vi "MU Acquire MtSync Data.vi"(6 "AnyThread? (F)":bool, 8 "error in (no error)":errorcluster, 10 "numberOfSamples":u64, 11 "MUhandle":u64) -> (0 "error out (no error)":errorcluster, 2 "data":T1(array[cluster]), 3 "function return":u32)   [LabVIEW 2017, in "MU_3SL_interface.lvlib"]
uses:
  MU_3SL_interface.lvlib
  lib/MU_3SL_interface.dll
panel:
  in  "data":T2
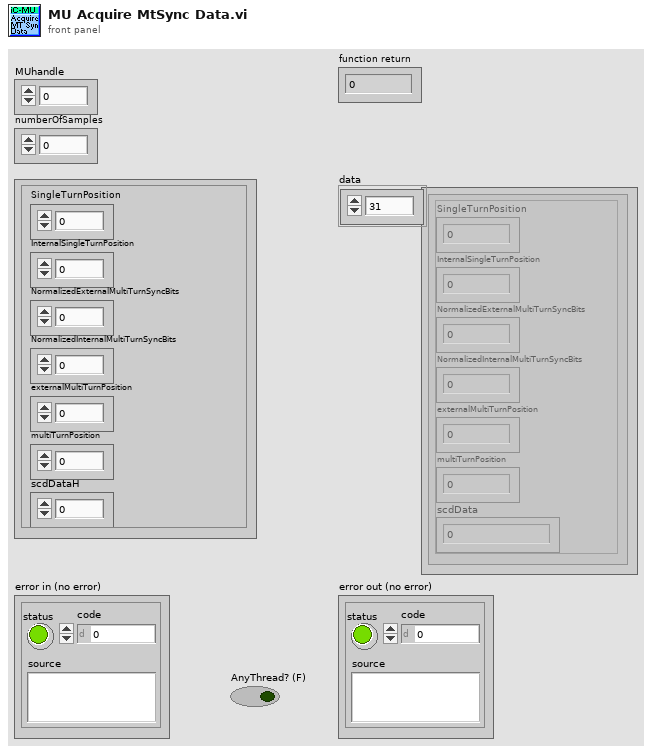
[diagram p1: front panel]
types:
  T1 = cluster{"SingleTurnPosition":u32, "InternalSingleTurnPosition":u32, "NormalizedExternalMultiTurnSyncBits":u32, "NormalizedInternalMultiTurnSyncBits":u32, "externalMultiTurnPosition":u32, "multiTurnPosition":u32, "scdData":u64}[]
  T2 = cluster{"SingleTurnPosition":u32, "InternalSingleTurnPosition":u32, "NormalizedExternalMultiTurnSyncBits":u32, "NormalizedInternalMultiTurnSyncBits":u32, "externalMultiTurnPosition":u32, "multiTurnPosition":u32, "scdDataH":u64}
  T3 = cluster{"SingleTurnPosition":u32, "InternalSingleTurnPosition":u32, "NormalizedExternalMultiTurnSyncBits":u32, "NormalizedInternalMultiTurnSyncBits":u32, "externalMultiTurnPosition":u32, "multiTurnPosition":u32, "scdDataH":u64}[]
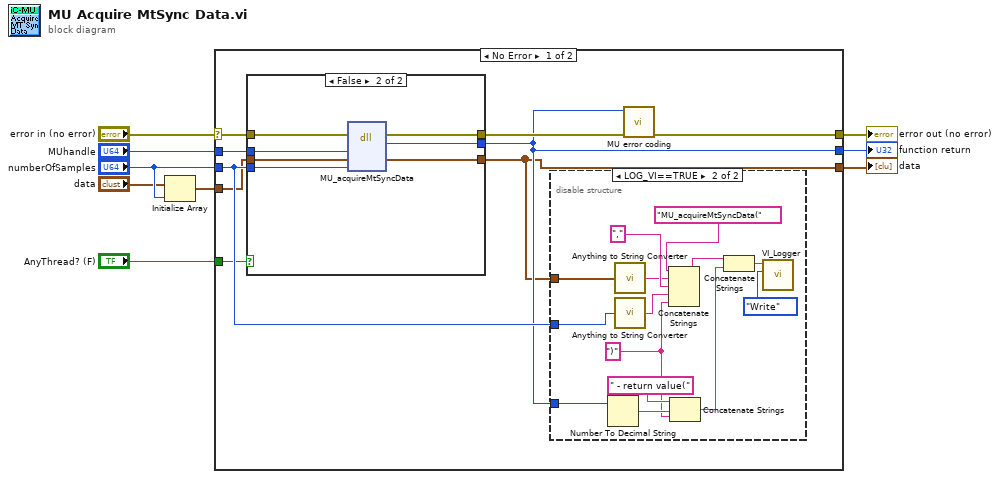
[diagram p0: block diagram]
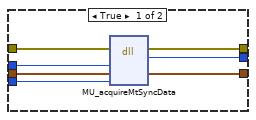
[diagram p2: hidden frame]
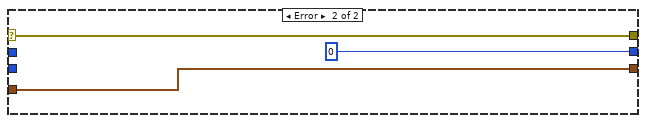
[diagram p4: hidden frame]
diagram:
  n1 = Initialize Array("data", "numberOfSamples") -> (w3:T3)
  n2 = case shown="No Error" "error in (no error)" {
    selector: "error in (no error)" -> [w15 w49]
    tunnel: [w13 u32 0] -> w9
    tunnel: "MUhandle" -> [w18 _]
    tunnel: [w16 w49] -> w7
    tunnel: "numberOfSamples" -> [w14 _]
    tunnel: w3 -> [w11 w47]
    tunnel: [w10 w47] -> w2
    tunnel: "AnyThread? (F)" -> [w12 _]
    frame No Error {
      n3 = case shown="False" w12 {
        tunnel: w18 -> [w25 w32]
        tunnel: [w24 w31] -> w17
        tunnel: w15 -> [w23 w30]
        tunnel: w11 -> [w22 w29]
        tunnel: w14 -> [w21 w28]
        tunnel: [w20 w27] -> w13
        tunnel: [w19 w26] -> w10
        frame True {
          n4 = dll-call lib="C:/Users/bes/AppData/Roaming/work/mu_9so/icsubmodules/soft_mu_3sl_master/lv_interface/lib/MU_3SL_interface**.*" fn="MU_acquireMtSyncData"(error in=w23, "MUhandle"=w25, "data"=w22, "numberOfSamples"=w21) -> (error out=w24:errorcluster, "return type"=w20:u32, "data"=w19:T3)  [unwired: 4 in, 1 out]
        }
        frame False {
          n5 = dll-call lib="C:/Users/bes/AppData/Roaming/work/mu_9so/icsubmodules/soft_mu_3sl_master/lv_interface/lib/MU_3SL_interface**.*" fn="MU_acquireMtSyncData"(error in=w30, "MUhandle"=w32, "data"=w29, "numberOfSamples"=w28) -> (error out=w31:errorcluster, "return type"=w27:u32, "data"=w26:T3)  [unwired: 4 in, 1 out]
        }
      }
      n6 = disable-structure shown="LOG_VI==TRUE" {
        disable-tunnel: w13 -> [_ w44]
        disable-tunnel: w14 -> [_ w36]
        disable-tunnel: w10 -> [_ w34]
        frame condition #0 {
        }
        frame condition #1 (active) {
          w37 = ")" ("string")
          n7 = Number To Decimal String(number=w44) -> (decimal integer string=w43:string)  [unwired: 1 in]
          n8 = call "Anything to String Converter.vi"("anything"=w34) -> ("String"=w33:string)
          n9 = call "Anything to String Converter.vi"("anything"=w36) -> ("String"=w35:string)
          n10 = Concatenate Strings("MU_acquireMtSyncData(" ("Info in"), w33, "," ("string"), w35, w37) -> (w42:string)
          n11 = Concatenate Strings(" - return value(" ("string"), w43, w37) -> (w41:string)
          n12 = Concatenate Strings(w42, w41) -> (w40:string)
          n13 = call "VI_Logger.vi"("Action (Read)"=enum16{"Write", "Read"}."Write", "Info in"=w40) -> ()  [unwired: 8 in, 2 out]
        }
      }
      n14 = call "MU error coding.vi"("error in (no error)"=w17, "function return in"=w13) -> ("error out"=w16:errorcluster)  [unwired: 9 in]
    }
    frame Error {
    }
  }
  "function return" <- w9
  "error out (no error)" <- w7
  "data" <- w2
